vi "FTW-Socket-Receive.vi"(0 "FTW Socket":refnum<class "FTW-Socket.lvclass">, 5 "Timeout":i32=100 format="%dmsec", 11 "error in":errorcluster) -> (4 "FTW Socket out":refnum<class "FTW-Socket.lvclass">, 6 "Message":string, 8 "Timed out?":bool, 15 "error out":errorcluster)   [LabVIEW 2013, in "FTW-Socket.lvclass"]
uses:
  FTW-Socket.lvclass
  FTW-Socket.lvclass/FTW-Socket.ctl
  error/FTW-ERR-ThrowGenericError.vi
  error/FTW-ERR-ThrowError.vi
  error/FTW-ERR-NoErrorConstant.vi
  error/FTW-ERR-CallChain.vi
  string/FTW-STR-ReplaceWhitespace.vi
panel:
  # "Inputs"
  # "Outputs"
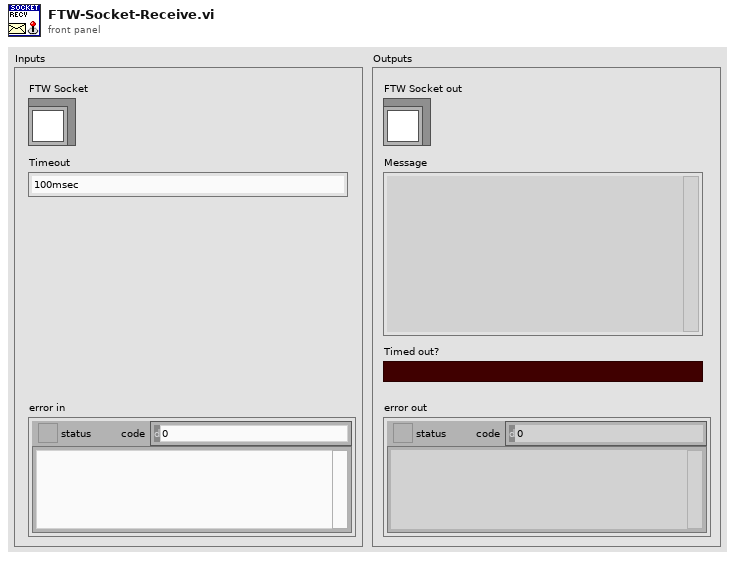
[diagram p1: front panel]
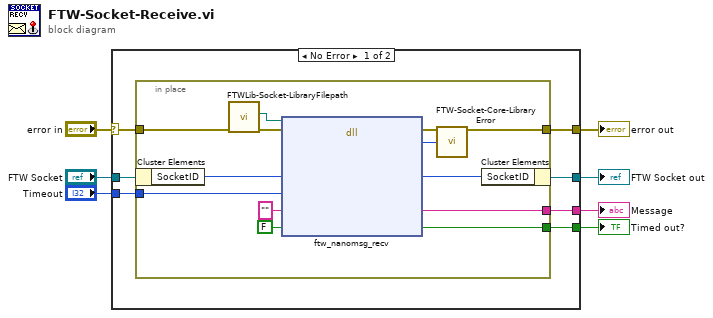
[diagram p0: block diagram]
diagram:
  n1 = case shown="No Error" "error in" {
    selector: "error in" -> [w11 w28]
    tunnel: "FTW Socket" -> [w14 w29]
    tunnel: [w13 w28] -> w3
    tunnel: [w12 w29] -> w4
    tunnel: "Timeout" -> [w10 _]
    tunnel: [w9 _] -> w1
    tunnel: [w8 _] -> w2
    frame No Error {
      n2 = in-place {
        in-place-border: w11 -> [w27]
        in-place-border: [w23] -> w13
        in-place-border: [w22] -> w9
        in-place-border: w10 -> [w16]
        in-place-border: [w18] -> w8
        n3 = in-place-cluster #1(w14) -> ("SocketID"=w25:i64)
        n4 = call "FTWLib-Socket-LibraryFilepath.vi"("error in"=w27) -> ("error out"=w20:errorcluster, "Library Filepath"=w21:path)  [unwired: 8 in, 1 out]
        n5 = dll-call lib="?" fn="ftw_nanomsg_recv"(path in=w21, error in=w20, "SocketID"=w25, "Timeout"=w16, "Incoming Msg"="", "Timed out?"=FALSE) -> (error out=w26:errorcluster, "Return Value"=w19:i64, "SocketID"=w24:i64, "Incoming Msg"=w18:string, "Timed out?"=w22:bool)  [unwired: 4 in, 1 out]
        n6 = call "FTW-Socket-Core-LibraryError.vi"("error in"=w26, "Return Value"=w19) -> ("error out"=w23:errorcluster)  [unwired: 13 in]
        n7 = in-place-cluster #1("SocketID"=w24) -> (w12:refnum<class "FTW-Socket.lvclass">)
      }
    }
    frame Error {
    }
  }
  "error out" <- w3
  "FTW Socket out" <- w4
  "Timed out?" <- w1
  "Message" <- w2
